vi "OffsetRect by Point Array and Rect.vi"(8 "错误输入":errorcluster, 10 "Points Array":cluster{"x":i16, "y":i16}[](array[cluster]), 11 "rect":T2 caption="矩形") -> (0 "错误输出":errorcluster, 3 "OffsetRect Array":T1(array[cluster]))   [LabVIEW 2012, in "Rect Tools.lvlib"]
uses:
  Rect Tools.lvlib
  OffsetRect by Point and Rect.vi
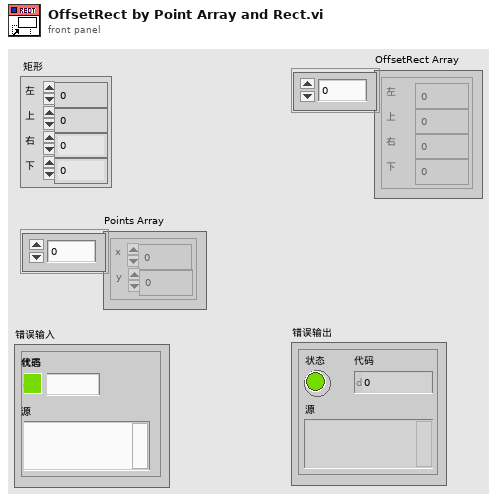
[diagram p1: front panel]
types:
  T1 = cluster{"left":i16, "top":i16, "right":i16, "bottom":i16}[]
  T2 = cluster{"left":i16, "top":i16, "right":i16, "bottom":i16}
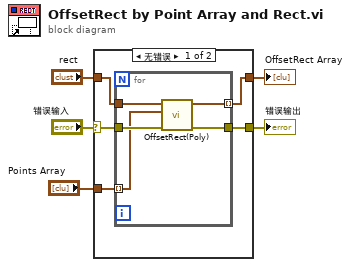
[diagram p0: block diagram]
diagram:
  n1 = case shown="无错误" "错误输入" {
    selector: "错误输入" -> [w7 w16]
    tunnel: [w6 w16] -> w4
    tunnel: "rect" -> [w9 _]
    tunnel: [w8 _] -> w1
    tunnel: "Points Array" -> [w10 _]
    frame No Error {
      n2 = for {
        tunnel: w10 -> [w11] mode=indexing
        tunnel: w9 -> [w15]
        tunnel: [w14] -> w8 mode=indexing
        tunnel: w7 -> [w13]
        tunnel: [w12] -> w6
        n3 = call-poly "OffsetRect(Poly).vi"("错误输入"=w13, "point"=w11, "rect"=w15) -> ("错误输出"=w12:errorcluster, "offset rect"=w14:T2)  [unwired: 7 in]
      }
    }
    frame Error {
    }
  }
  "错误输出" <- w4
  "OffsetRect Array" <- w1
